vi "Initialise SSH Client.vi"(8 "error in (no error)":errorcluster, 11 "Connection Info":T2={"host IP"="", "port"=22, "username"="lanforge", "password"="lanforge", "Connection Name"=""}) -> (0 "error out":errorcluster, 2 "References":T1)   [LabVIEW 2017, in "SSH.lvlib"]
doc: "Creates a new SSH client and connects to it with the requested parameters"
uses:
  SSH.lvlib
  Connection Info.ctl
  dotNET references.ctl
  C:/Users/ukhornp/Documents/SSH/References/Renci.SshNet.dll
  References/Renci.SshNet.dll
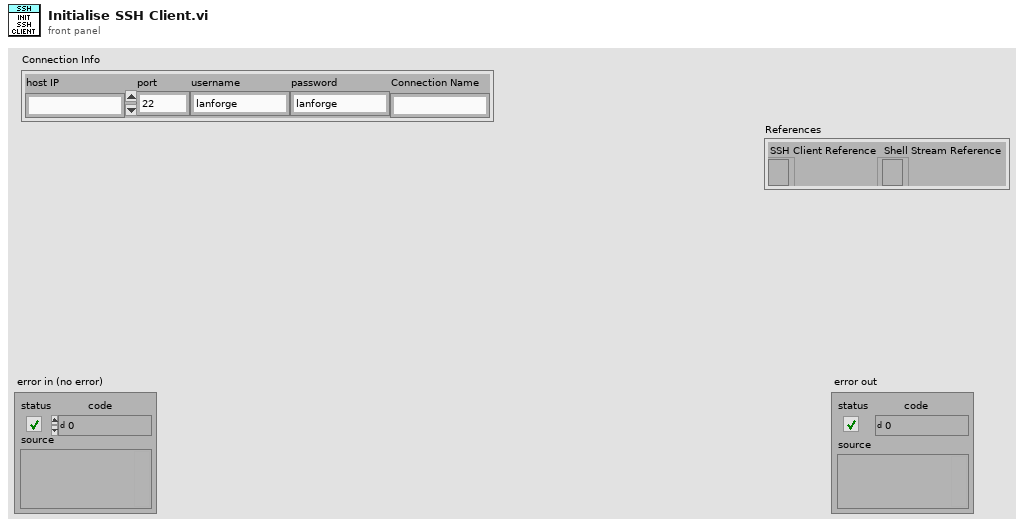
[diagram p1: front panel]
types:
  T1 = typedef "SSH.lvlib/dotNET references.ctl" = cluster{"SSH Client Reference":refnum<k24>, "Shell Stream Reference":refnum<k24>}
  T2 = typedef "SSH.lvlib/Connection Info.ctl" = cluster{"host IP":string, "port":i32, "username":string, "password":string, "Connection Name":string}
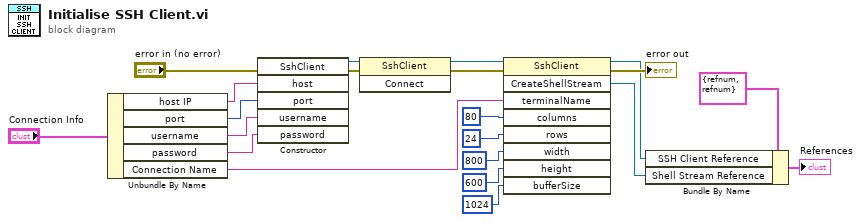
[diagram p0: block diagram]
diagram:
  n1 = Unbundle By Name("Connection Info") -> ("host IP"=w12:string, "port"=w11:i32, "username"=w10:string, "password"=w9:string, "Connection Name"=w8:string)
  n2 = constructor class="SshClient"(error in="error in (no error)", "host"=w12, "port"=w11, "username"=w10, "password"=w9) -> (reference out=w13:refnum<k24>, error out=w14:errorcluster)  [unwired: 2 in, 5 out]
  n3 = invoke class="SshClient" method="Connect"(reference=w13, error in=w14) -> (reference out=w15:refnum<k24>, error out=w16:errorcluster)  [unwired: 1 in, 1 out]
  n4 = invoke class="SshClient" method="CreateShellStream"(reference=w15, error in=w16, "terminalName"=w8, "columns"=u32 80, "rows"=u32 24, "width"=u32 800, "height"=u32 600, "bufferSize"=1024) -> (reference out=w3:refnum<k24>, error out=→"error out":errorcluster, "CreateShellStream"=w2:refnum<k24>)  [unwired: 1 in, 6 out]
  n5 = Bundle By Name(cluster=T1 {"SSH Client Reference"=refnum, "Shell Stream Reference"=refnum} ("References"), "SSH Client Reference"=w3, "Shell Stream Reference"=w2) -> (→"References":T1)
